vi "Find F-I.vi"(8 "error in (no error)":errorcluster, 9 "Tag":string, 10 "Abs_Value In":refnum<class "Abs_Value.lvclass">, 11 "Fault-Injection Bus in":refnum<class "Fault-Injection Bus.lvclass">) -> (0 "error out":errorcluster, 1 "Updated Tag":bool, 2 "Abs_Value Out":refnum<class "Abs_Value.lvclass">, 3 "Fault-Injection Bus out":refnum<class "Fault-Injection Bus.lvclass">)   [LabVIEW 2021, in "Fault-Injection Bus.lvclass"]
uses:
  Fault-Injection Bus.lvclass
  <vilib>/TSA/Abstract Data Classes/Abs_Types/Value/Abs_Value.lvclass
  C:/Program Files (x86)/National Instruments/LabVIEW 2021/vi.lib/TSA/Abstract Data Classes/Abs_Types/Type/Abs_Type.lvclass
  <vilib>/TSA/Abstract Data Classes/Abs_Types/Type/Abs_Type.lvclass/Abs_Type.ctl
  Fault-Injection Bus.lvclass/Fault-Injection Bus.ctl
  Properties/Read F-I Map.vi
  Omni-Bus/Omni_Bus.lvclass
  <vilib>/TSA/Abstract Data Classes/Abs_Types/Type/Abs_Type.lvclass
  C:/Program Files (x86)/National Instruments/LabVIEW 2021/vi.lib/TSA/Abstract Data Classes/Abs_Types/Value/Abs_Value.lvclass
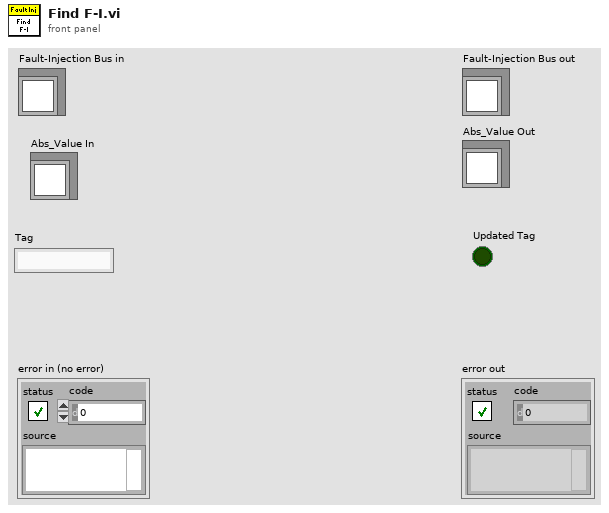
[diagram p1: front panel]
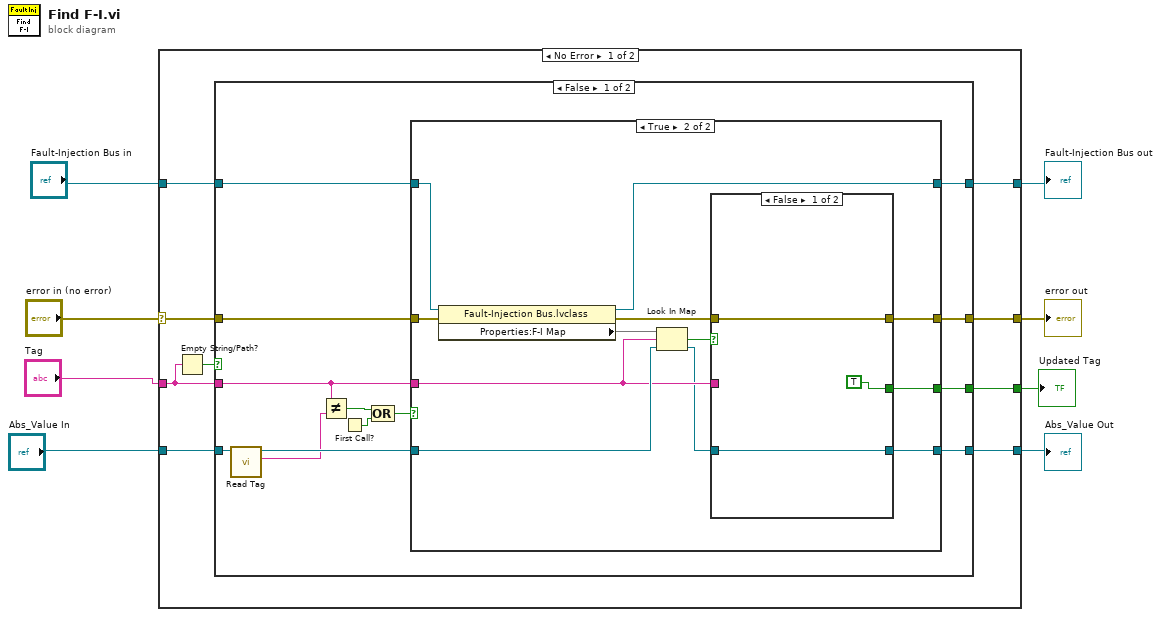
[diagram p0: block diagram]
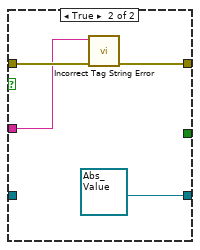
[diagram p3: hidden frame]
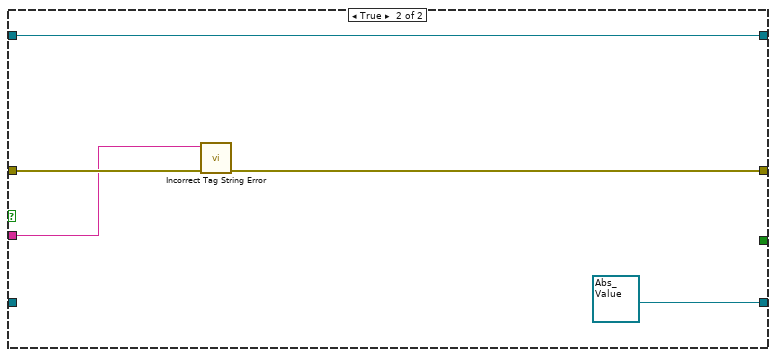
[diagram p4: hidden frame]
diagram:
  n1 = case shown="No Error" "error in (no error)" {
    selector: "error in (no error)" -> [w17 w60]
    tunnel: [w14 w60] -> w4
    tunnel: [w13 w59] -> w5
    tunnel: "Fault-Injection Bus in" -> [w16 w59]
    tunnel: "Tag" -> [w11 _]
    tunnel: [w15 w58] -> w2
    tunnel: "Abs_Value In" -> [w12 w58]
    tunnel: [w9 _] -> w1
    frame No Error {
      n2 = Empty String/Path?(string/path=w11) -> (empty?=w10:bool)
      n3 = case shown="False" w10 {
        tunnel: w17 -> [w30 w56]
        tunnel: w16 -> [w29 w57]
        tunnel: [w28 refnum<class "Abs_Value.lvclass"> refnum ("Abs_Value.lvclass")] -> w15
        tunnel: [w27 w55] -> w14
        tunnel: [w26 w57] -> w13
        tunnel: w11 -> [w22 w54]
        tunnel: w12 -> [w21 _]
        tunnel: [w18 _] -> w9
        frame False {
          n4 = call <vilib>:"Read Tag.vi"("Abs_Type in"=w21) -> ("Tag"=w19:string, "Abs_Type out"=w20:refnum<class "Abs_Value.lvclass">)  [unwired: 9 in]
          n5 = Not Equal?(x=w22, y=w19) -> (x != y?=w25:bool)
          n6 = First Call?() -> (First Call?: T/F=w23:bool)
          n7 = Compound Arithmetic op=OR(w25, w23) -> (w24:bool)
          n8 = case shown="True" w24 {
            tunnel: w30 -> [w32 w45]
            tunnel: w29 -> [w31 w44]
            tunnel: [w33 w35] -> w28
            tunnel: [w32 w39] -> w27
            tunnel: [w31 w42] -> w26
            tunnel: w20 -> [w33 w41]
            tunnel: w22 -> [_ w38]
            tunnel: [_ w34] -> w18
            frame False {
            }
            frame True {
              n9 = property class="Fault-Injection Bus.lvclass"(reference=w44, error in=w45) -> (reference out=w42:refnum<class "Fault-Injection Bus.lvclass">, error out=w40:errorcluster, "Properties:F-I Map"=w43:map{string, refnum<class "Abs_Value.lvclass">})
              n10 = Look In Map(map=w43, key=w38, default value=w41) -> (key not found?=w37:bool, value=w36:refnum<class "Abs_Value.lvclass">)
              n11 = case shown="False" w37 {
                tunnel: w40 -> [w48 w52]
                tunnel: [w48 w51] -> w39
                tunnel: w38 -> [_ w50]
                tunnel: w36 -> [w47 _]
                tunnel: [w47 refnum<class "Abs_Value.lvclass"> refnum ("Abs_Value.lvclass")] -> w35
                tunnel: [TRUE _] -> w34
                frame False {
                }
                frame True {
                  n12 = call "Incorrect Tag String Error.vi"("error in (no error)"=w52, "Tag"=w50) -> ("error out"=w51:errorcluster)  [unwired: 9 in]
                }
              }
            }
          }
        }
        frame True {
          n13 = call "Incorrect Tag String Error.vi"("error in (no error)"=w56, "Tag"=w54) -> ("error out"=w55:errorcluster)  [unwired: 9 in]
        }
      }
    }
    frame Error {
    }
  }
  "error out" <- w4
  "Fault-Injection Bus out" <- w5
  "Abs_Value Out" <- w2
  "Updated Tag" <- w1
